vi "Pack Return Message Adapter.vi"(9 "Return Priority (Normal)":T1=enum."Normal", 10 "Return Enqueuer":refnum<class "Message Enqueuer.lvclass">, 11 "Return Message":refnum<class "Message.lvclass">) -> (3 "ReturnMessageAdapter Out":refnum<class "ReturnMessageAdapter.lvclass">)   [LabVIEW 2020, in "ReturnMessageAdapter.lvclass"]
doc: "包装返回消息适配器"
uses:
  ReturnMessageAdapter.lvclass
  <vilib>/ActorFramework/Message Enqueuer/Message Enqueuer.lvclass
  <vilib>/ActorFramework/Message Enqueuer/Message Priority.ctl
  <vilib>/ActorFramework/Message/Message.lvclass
  ReturnMessageAdapter.lvclass/ReturnMessageAdapter.ctl
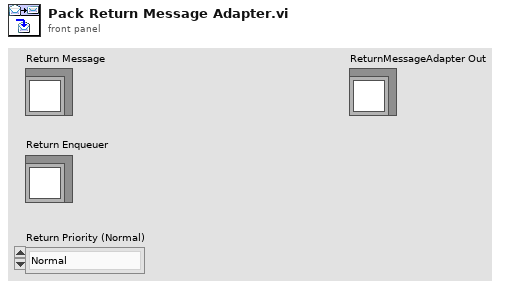
[diagram p1: front panel]
types:
  T1 = typedef "Actor Framework.lvlib/Message Enqueuer.lvclass/Message Priority.ctl" = enum16{"Low", "Normal", "High"}
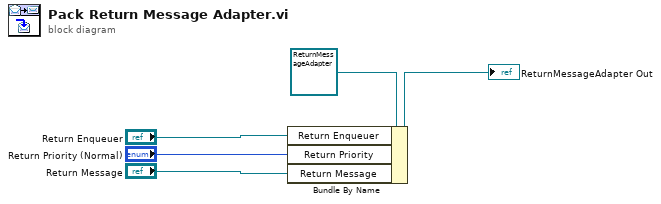
[diagram p0: block diagram]
diagram:
  n1 = Bundle By Name(cluster=refnum<class "ReturnMessageAdapter.lvclass"> refnum ("ReturnMessageAdapter In"), "Return Enqueuer"="Return Enqueuer", "Return Priority"="Return Priority (Normal)", "Return Message"="Return Message") -> (→"ReturnMessageAdapter Out":refnum<class "ReturnMessageAdapter.lvclass">)
